vi "Init Actor Core.vi"(8 "error in (no error)":errorcluster, 11 "Monitor Controller in":refnum<class "Monitor Controller.lvclass">) -> (0 "error out":errorcluster, 3 "Monitor Controller out":refnum<class "Monitor Controller.lvclass">)   [LabVIEW 2015, in "Monitor Controller.lvclass"]
uses:
  Monitor Controller.lvclass
  Measurements/Timer/Timer.lvclass
  Monitor Controller.lvclass/Monitor Controller.ctl
  Measure Controller/Measure Controller.lvclass/Measure Controller.ctl
  Measure Controller/Write File prefix.vi
  Measure Controller/Measure Controller.lvclass
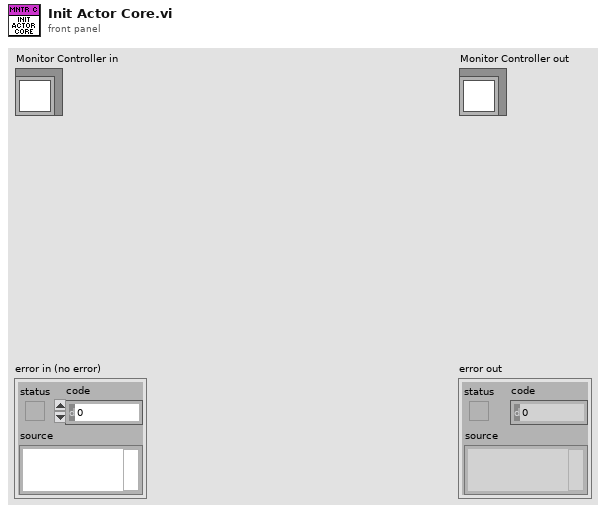
[diagram p1: front panel]
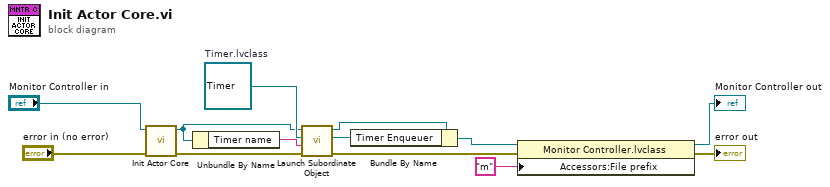
[diagram p0: block diagram]
diagram:
  w11 = refnum<class "Timer.lvclass"> refnum  # Timer.lvclass
  n1 = call-parent "Init Actor Core.vi"("error in (no error)"="error in (no error)", "Measure Object in"="Monitor Controller in") -> ("error out"=w8:errorcluster, "Measure Object out"=w10:refnum<class "Monitor Controller.lvclass">)  [unwired: 8 in]
  n2 = Unbundle By Name(w10) -> ("Timer name"=w9:string)
  n3 = call-dynamic "Launch Subordinate Object.vi"("error in (no error)"=w8, "Name"=w9, "Subordinate Object"=w11, "Measure Object in"=w10) -> ("error out"=w2:errorcluster, "Nested Actor's Enqueuer"=w6:refnum<class "Message Enqueuer.lvclass">, "Measure Object out"=w7:refnum<class "Monitor Controller.lvclass">)  [unwired: 5 in]
  n4 = Bundle By Name(cluster=w7, "Timer Enqueuer"=w6) -> (w5:refnum<class "Monitor Controller.lvclass">)
  n5 = property class="Monitor Controller.lvclass"(reference=w5, error in=w2, "Accessors:File prefix"="m" ("File prefix")) -> (reference out=→"Monitor Controller out":refnum<class "Monitor Controller.lvclass">, error out=→"error out":errorcluster)
